vi "Index.vi"(11 "Index?":bool) -> ()   [LabVIEW 2016]
uses:
  <vilib>/Rock Robotics/WPI/Relay/WPI_RelayValue.ctl
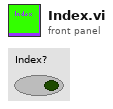
[diagram p1: front panel]
types:
  T1 = typedef "WPI_RelayValue.ctl" = enum16{"Off", "On", "Forward", "Reverse"}
  T2 = typedef "WPI_RelayDevRef.ctl" = cluster{"DevStatus":errorcluster, "Relay Channel":T3, "Relay Direction":T4}
  T3 = typedef "FPGA_DIORelayChannel.ctl" = enum8{"Relay 0", "Relay 1", "Relay 2", "Relay 3", "Invalid"}
  T4 = typedef "WPI_RelayDirection.ctl" = enum16{"Both directions", "Forward only", "Reverse only"}
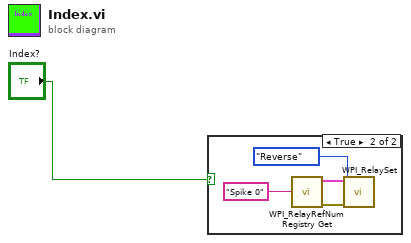
[diagram p0: block diagram]
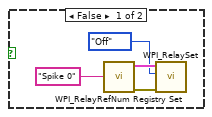
[diagram p2: hidden frame]
diagram:
  n1 = case shown="True" "Index?" {
    frame False {
      n2 = call <vilib>:"WPI_RelayRefNum Registry Set.vi"("refnum name"="Spike 0") -> ("error out"=w5:errorcluster, "RelayDevRef"=w4:T2)  [unwired: 9 in]
      n3 = call <vilib>:"WPI_RelaySet.vi"("error in (no error)"=w5, "RelayValue"=WPI_RelayValue."Off", "RelayDevRef"=w4) -> ()  [unwired: 7 in, 2 out]
    }
    frame True {
      n4 = call <vilib>:"WPI_RelayRefNum Registry Get.vi"("refnum name"="Spike 0") -> ("error out"=w9:errorcluster, "RelayDevRef"=w8:T2)  [unwired: 9 in]
      n5 = call <vilib>:"WPI_RelaySet.vi"("error in (no error)"=w9, "RelayValue"=WPI_RelayValue."Reverse", "RelayDevRef"=w8) -> ()  [unwired: 7 in, 2 out]
    }
  }
